vi "getLocalPath.vi"(8 "error in (no error)":errorcluster, 11 "ILogFileInfo in":refnum<class "ILogFileInfo.lvclass">) -> (0 "error out":errorcluster, 2 "Local Path out":string, 3 "ILogFileInfo out":refnum<class "ILogFileInfo.lvclass">)   [LabVIEW 2022 SP3, in "openDAQ.lvlib" / "IBaseObject.lvlib" / "ILogFileInfo.lvlib" / "ILogFileInfo.lvclass"]
uses:
  <instrlib>/openDAQ/Public/Classes/ILogFileInfo/ILogFileInfo.lvclass
  <instrlib>/openDAQ/Public/Classes/ILogFileInfo/ILogFileInfo.lvclass/ILogFileInfo.ctl
  <instrlib>/openDAQ/Public/Classes/daqCoreTypes/IString/IString.lvclass
  <instrlib>/openDAQ/Binaries/Windows/x86/copendaq32.dll
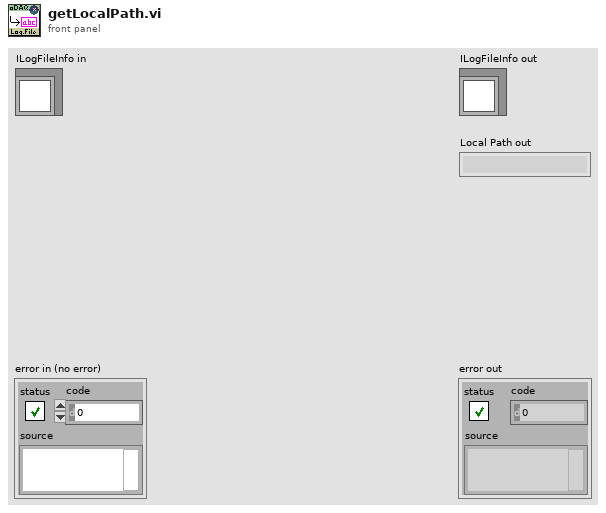
[diagram p1: front panel]
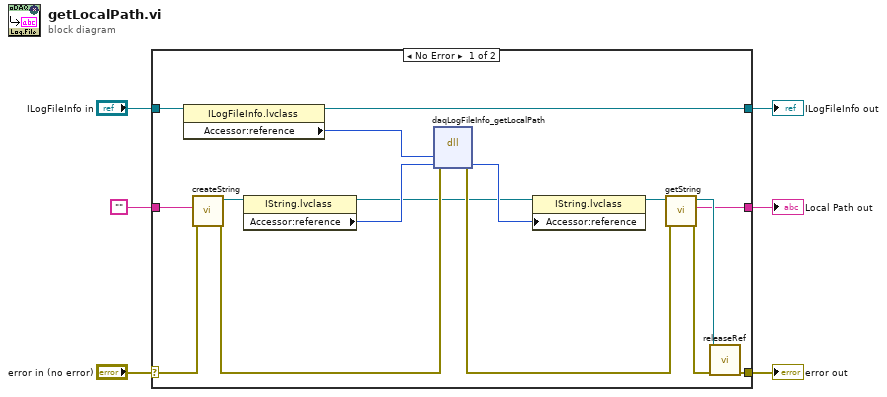
[diagram p0: block diagram]
diagram:
  n1 = case shown="No Error" "error in (no error)" {
    selector: "error in (no error)" -> [w8 w25]
    tunnel: [w11 w25] -> w5
    tunnel: [w17 w24] -> w3
    tunnel: "ILogFileInfo in" -> [w18 w24]
    tunnel: "" -> [w13 w23]
    tunnel: [w9 w23] -> w1
    frame No Error {
      n2 = property class="ILogFileInfo.lvclass"(reference=w18) -> (reference out=w17:refnum<class "ILogFileInfo.lvclass">, "Accessor:reference"=w12:i64)  [unwired: 1 in, 1 out]
      n3 = call <instrlib>:"createString.vi"("error in (no error)"=w8, "String"=w13) -> ("error out"=w22:errorcluster, "IString out"=w15:refnum<class "IString.lvclass">)  [unwired: 8 in]
      n4 = property class="IString.lvclass"(reference=w15) -> (reference out=w16:refnum<class "IString.lvclass">, "Accessor:reference"=w20:i64)  [unwired: 1 in, 1 out]
      n5 = dll-call lib="C:/Program Files (x86)/National Instruments/LabVIEW 2022/instr.lib/openDAQ/Binaries/Windows/x86/copendaq*.*" fn="daqLogFileInfo_getLocalPath"(error in=w22, "logFileInfo"=w12, "localPath"=w20) -> (error out=w21:errorcluster, "localPath"=w19:i64)  [unwired: 4 in, 1 out]
      n6 = property class="IString.lvclass"(reference=w16, "Accessor:reference"=w19) -> (reference out=w14:refnum<class "IString.lvclass">)  [unwired: 1 in, 1 out]
      n7 = call <instrlib>:"getString.vi"("error in (no error)"=w21, "IString in"=w14) -> ("error out"=w7:errorcluster, "String out"=w9:string, "IString out"=w10:refnum<class "IString.lvclass">)  [unwired: 7 in]
      n8 = call-dynamic "releaseRef.vi"("error in (no error)"=w7, "IBaseObject in"=w10) -> ("error out"=w11:errorcluster)  [unwired: 9 in]
    }
    frame Error {
    }
  }
  "error out" <- w5
  "ILogFileInfo out" <- w3
  "Local Path out" <- w1
